vi "Send Panel Close.vi"(6 "Name (use VI name)":string, 8 "Discarded?":bool, 9 "Time":u32, 10 "VI Refnum":refnum<vi>, 11 "Message Enqueuer in":refnum<class "Message Enqueuer.lvclass">) -> (0 "error out":errorcluster)   [LabVIEW 2015, in "ActorAutoRegistration.lvlib" / "PanelCloseMsg.lvclass"]
doc: "<License>\nCopyright © 2017 Composed Systems, LLC | All rights reserved\nwww.composed.io\n\nAuthor: Ethan Stern <ethan.stern@composed.io>\n\nThis software is provided \"AS IS\" WITHOUT WARRANTIES, either express or implied, AND IS FOR EDUCATIONAL PURPOSES ONLY.\n</License>"
uses:
  PanelCloseMsg.lvclass
  <vilib>/ActorFramework/Message Enqueuer/Message Enqueuer.lvclass
  <vilib>/ActorFramework/Message Enqueuer/Message Priority.ctl
  PanelCloseMsg.lvclass/PanelCloseMsg.ctl
  EventDataMessage/EventDataMessage.lvclass
panel:
  in  "error in (no error)":errorcluster
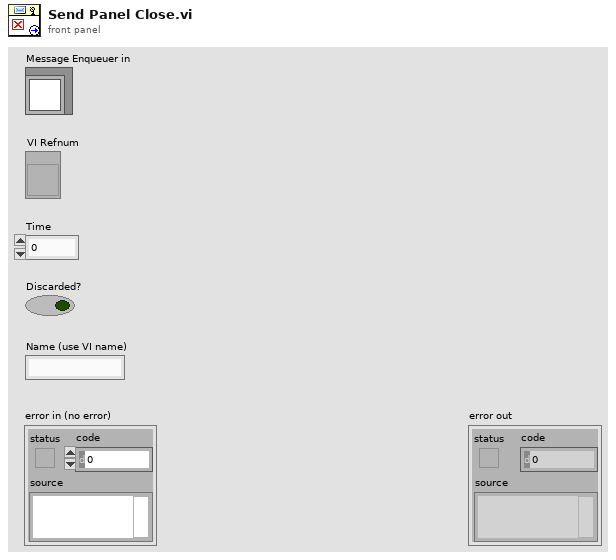
[diagram p1: front panel]
types:
  T1 = typedef "Actor Framework.lvlib/Message Enqueuer.lvclass/Message Priority.ctl" = enum16{"Low", "Normal", "High"}
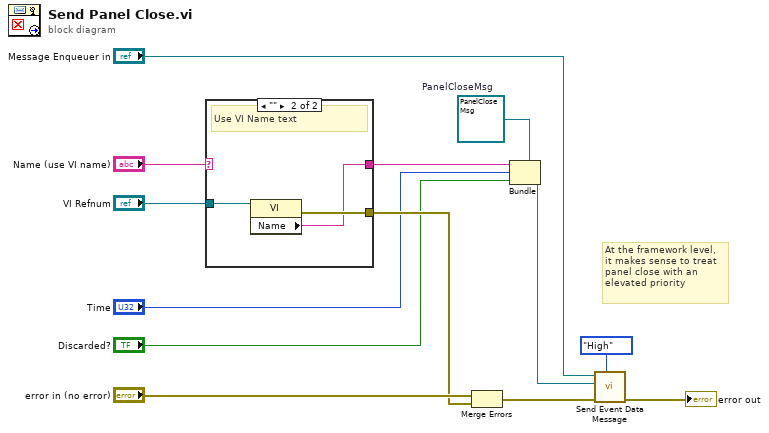
[diagram p0: block diagram]
diagram:
  w10 = refnum<class "PanelCloseMsg.lvclass"> refnum  # PanelCloseMsg
  # "At the framework level,\nit makes sense to treat\npanel close with an\nelevated priority"
  n1 = case shown="\"\"" "Name (use VI name)" {
    selector: "Name (use VI name)" -> [w14 _]
    tunnel: [w14 w15] -> w13
    tunnel: "VI Refnum" -> [_ w17]
    tunnel: [_ w16] -> w7
    frame Default {
      # "Use string provided"
    }
    frame "" {
      # "Use VI Name text"
      n2 = property class="VI"(reference=w17) -> (error out=w16:errorcluster, "Name"=w15:string)  [unwired: 1 in, 1 out]
    }
  }
  n3 = Merge Errors("error in (no error)", w7) -> (w8:errorcluster)
  n4 = Bundle(cluster=w10, w13, "Time", "Discarded?") -> (w5:refnum<class "PanelCloseMsg.lvclass">)
  n5 = call "Send Event Data Message.vi"("Message Priority (Normal)"=Message_Priority."High", "error in (no error)"=w8, "EventDataMessage in"=w5, "Message Enqueuer in"="Message Enqueuer in") -> ("error out"=→"error out":errorcluster)  [unwired: 7 in]
